vi "TSCAN Close.vi"(0 "路径输入":path, 11 "错误输入（无错误）":errorcluster) -> (4 "路径输出":path, 15 "错误输出":errorcluster)   [LabVIEW 2013]
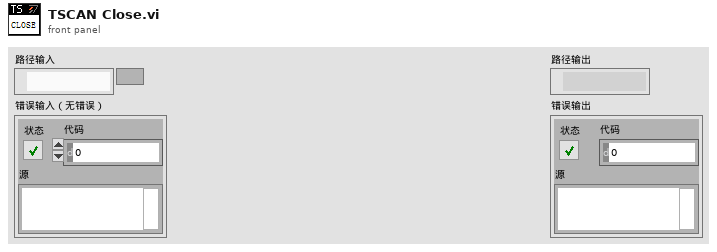
[diagram p1: front panel]
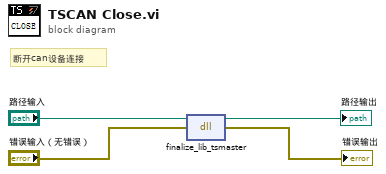
[diagram p0: block diagram]
diagram:
  # "断开can设备连接"
  n1 = dll-call lib="PTH1Habs CUsers\nAdministratorDesktopTS_Can通讯PathTSMaster.dll" fn="finalize_lib_tsmaster"(path in="路径输入", error in="错误输入（无错误）") -> (path out=→"路径输出":path, error out=→"错误输出":errorcluster)  [unwired: 2 in]
